vi "GetIndicatorData.vi"(0 "reference in":refnum<class "WebFrontPanel.lvclass">, 5 "error in (no error)":errorcluster) -> (14 "reference out":refnum<class "WebFrontPanel.lvclass">, 15 "String":string, 19 "error out":errorcluster)   [LabVIEW 2014, in "WebFrontPanel.lvclass"]
uses:
  WebFrontPanel.lvclass
  Object_class/Object.lvclass
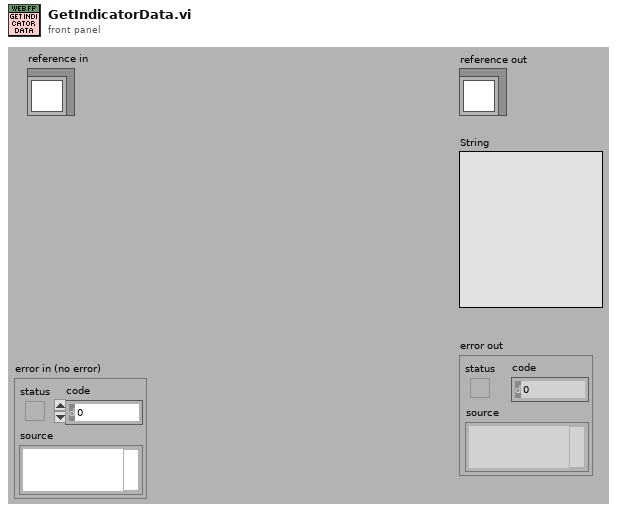
[diagram p1: front panel]
types:
  T1 = typedef "WebFrontPanel.lvclass/ObjectAttributes.ctl" = cluster{"VI Name":string, "VI Reference":refnum<vi>, "Queue To VI ":refnum<queue>, "Controls":refnum<class "Object.lvclass">[], "Indicators":refnum<class "Object.lvclass">[], "Decorations":refnum<class "Object.lvclass">[]}
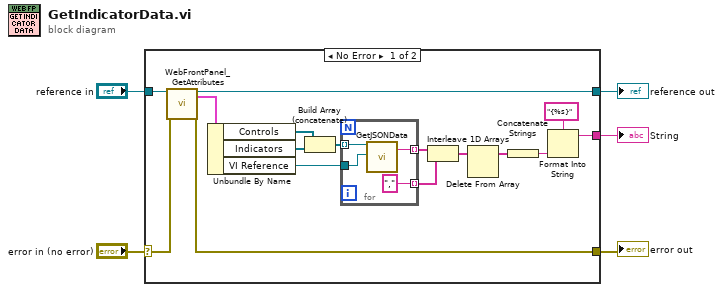
[diagram p0: block diagram]
diagram:
  n1 = case shown="No Error" "error in (no error)" {
    selector: "error in (no error)" -> [w21 w27]
    tunnel: [w19 w27] -> w4
    tunnel: [w17 w26] -> w2
    tunnel: "reference in" -> [w18 w26]
    tunnel: [w9 _] -> w1
    frame No Error {
      n2 = call "WebFrontPanel_GetAttributes.vi"("reference in"=w18, "error in (no error)"=w21) -> ("reference out"=w17:refnum<class "WebFrontPanel.lvclass">, "Data"=w20:T1, "error out"=w19:errorcluster)  [unwired: 14 in, 1 out]
      n3 = Unbundle By Name(w20) -> ("Controls"=w8:refnum<class "Object.lvclass">[], "Indicators"=w7:refnum<class "Object.lvclass">[], "VI Reference"=w16:refnum<vi>)
      n4 = Build Array (concatenate)(w8, w7) -> (w6:refnum<class "Object.lvclass">[])
      n5 = for {
        tunnel: w6 -> [w25] mode=indexing
        tunnel: w16 -> [w22]
        tunnel: [w24] -> w15 mode=indexing
        tunnel: [","] -> w14 mode=indexing
        n6 = call-dynamic "GetJSONData.vi"("reference in"=w25, "VI Reference"=w22) -> ("JSON string"=w24:string)  [unwired: 15 in, 2 out]
      }
      n7 = Interleave 1D Arrays(w15, w14) -> (w13:string[])
      n8 = Delete From Array(array=w13) -> (array with subset deleted=w12:string[])  [unwired: 2 in, 1 out]
      n9 = Concatenate Strings(w12) -> (w11:string)
      n10 = Format Into String(format string="{%s}", w11) -> (resulting string=w9:string)  [unwired: 2 in, 1 out]
    }
    frame Error {
    }
  }
  "error out" <- w4
  "reference out" <- w2
  "String" <- w1
